vi "niTuner Get Attenuation.vi"(8 "error in":errorcluster, 11 "taskID in":i32 format="%.0x") -> (0 "error out":errorcluster, 1 "scale factor":dbl format="%.2f", 2 "attenuation":dbl format="%.2f", 3 "taskID out":i32 format="%.0x")   [LabVIEW 2011]
doc: "This VI returns the IF signal attenuation for each frequency in the scan list."
uses:
  nipxi5600u.dll
panel:
  in  "List Size":u32=1 min=1 max=1
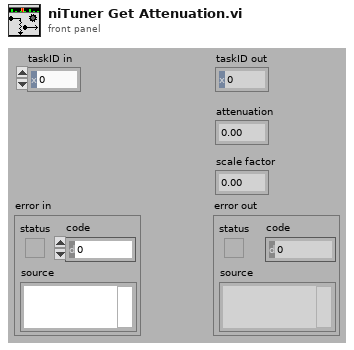
[diagram p1: front panel]
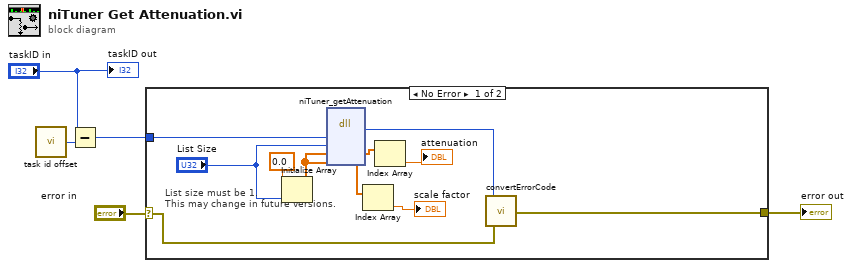
[diagram p0: block diagram]
diagram:
  n1 = call <instrlib>:"task id offset.vi"() -> ("taskID offset"=w2:i32)
  n2 = Subtract(x="taskID in", y=w2) -> (x-y=w3:i32)
  n3 = case shown="No Error" "error in" {
    selector: "error in" -> [w10 w17]
    tunnel: [w8 w17] -> w4
    tunnel: w3 -> [w16 _]
    frame No Error {
      # "List size must be 1.\nThis may change in future versions."
      n4 = Initialize Array(0.0 ("Element Data"), "List Size") -> (w11:dbl[])
      n5 = dll-call lib="nipxi5600u.dll" fn="niTuner_getAttenuation"("taskID"=w16, "listSize"="List Size", "attenuation"=w11, "scaleFactor"=w11) -> (w9:i32, "attenuation"=w15:dbl[], "scaleFactor"=w14:dbl[])  [unwired: 5 in, 2 out]
      n6 = Index Array(array=w14) -> (element=→"scale factor":dbl)  [unwired: 1 in]
      n7 = Index Array(array=w15) -> (element=→"attenuation":dbl)  [unwired: 1 in]
      n8 = call <instrlib>:"convertErrorCode.vi"("error in"=w10, "error code"=w9) -> ("error out"=w8:errorcluster)
    }
    frame Error {
    }
  }
  "error out" <- w4
  "taskID out" <- "taskID in"
